vi "_old_Load_SetList_SubVI_v4.1.vi"(0 "Path":path) -> (1 "Procedure Name":string="IBS_PICameraTest_29Sep04", 2 "Paramaters":T1={"Master PB Staging List"=[{"Output Bits"=[], "Delay (s)"="", "String"="", "Halt?"=FALSE}, {"Output Bits"=[], "Delay (s)"="", "String"="", "Halt?"=FALSE}, {"Output Bits"=[], "Delay (s)"="", "String"="", "Halt?"=FALSE}, {"Output Bits"=[], "Delay (s)"="", "String"="", "Halt?"=FALSE}, {"Output Bits"=[], "Delay (s)"="", "String"="", "Halt?"=FALSE}, {"Output Bits"=[], "Delay (s)"="", "String"="", "Halt?"=FALSE}, {"Output Bits"=[], "Delay (s)"="", "String"="", "Halt?"=FALSE}, {"Output Bits"=[], "Delay (s)"="", "String"="", "Halt?"=FALSE}, {"Output Bits"=[], "Delay (s)"="", "String"="", "Halt?"=FALSE}, {"Output Bits"=[], "Delay (s)"="", "String"="", "Halt?"=FALSE}, {"Output Bits"=[], "Delay (s)"="", "String"="", "Halt?"=FALSE}, {"Output Bits"=[], "Delay (s)"="", "String"="", "Halt?"=FALSE}, {"Output Bits"=[], "Delay (s)"="", "String"="", "Halt?"=FALSE}, {"Output Bits"=[], "Delay (s)"="", "String"="", "Halt?"=FALSE}, {"Output Bits"=[], "Delay (s)"="", "String"="", "Halt?"=FALSE}, {"Output Bits"=[], "Delay (s)"="", "String"="", "Halt?"=FALSE}, {"Output Bits"=[], "Delay (s)"="", "String"="", "Halt?"=FALSE}, {"Output Bits"=[], "Delay (s)"="", "String"="", "Halt?"=FALSE}, {"Output Bits"=[], "Delay (s)"="", "String"="", "Halt?"=FALSE}, {"Output Bits"=[], "Delay (s)"="", "String"="", "Halt?"=FALSE}, {"Output Bits"=[], "Delay (s)"="", "String"="", "Halt?"=FALSE}, {"Output Bits"=[], "Delay (s)"="", "String"="", "Halt?"=FALSE}, {"Output Bits"=[], "Delay (s)"="", "String"="", "Halt?"=FALSE}, {"Output Bits"=[], "Delay (s)"="", "String"="", "Halt?"=FALSE}, {"Output Bits"=[], "Delay (s)"="", "String"="", "Halt?"=FALSE}, {"Output Bits"=[], "Delay (s)"="", "String"="", "Halt?"=FALSE}, {"Output Bits"=[], "Delay (s)"="", "String"="", "Halt?"=FALSE}, {"Output Bits"=[], "Delay (s)"="", "String"="", "Halt?"=FALSE}, {"Output Bits"=[], "Delay (s)"="", "String"="", "Halt?"=FALSE}, {"Output Bits"=[], "Delay (s)"="", "String"="", "Halt?"=FALSE}, {"Output Bits"=[], "Delay (s)"="", "String"="", "Halt?"=FALSE}, {"Output Bits"=[], "Delay (s)"="", "String"="", "Halt?"=FALSE}, {"Output Bits"=[], "Delay (s)"="", "String"="", "Halt?"=FALSE}, {"Output Bits"=[], "Delay (s)"="", "String"="", "Halt?"=FALSE}, {"Output Bits"=[], "Delay (s)"="", "String"="", "Halt?"=FALSE}, {"Output Bits"=[], "Delay (s)"="", "String"="", "Halt?"=FALSE}, {"Output Bits"=[], "Delay (s)"="", "String"="", "Halt?"=FALSE}, {"Output Bits"=[], "Delay (s)"="", "String"="", "Halt?"=FALSE}, {"Output Bits"=[], "Delay (s)"="", "String"="", "Halt?"=FALSE}, {"Output Bits"=[], "Delay (s)"="", "String"="", "Halt?"=FALSE}, {"Output Bits"=[], "Delay (s)"="", "String"="", "Halt?"=FALSE}, {"Output Bits"=[], "Delay (s)"="", "String"="", "Halt?"=FALSE}, {"Output Bits"=[], "Delay (s)"="", "String"="", "Halt?"=FALSE}, {"Output Bits"=[], "Delay (s)"="", "String"="", "Halt?"=FALSE}], "Slave PB Staging List"=[{"Output Bits"=[], "Delay (s)"="", "String"="", "Halt?"=FALSE}, {"Output Bits"=[], "Delay (s)"="", "String"="", "Halt?"=FALSE}, {"Output Bits"=[], "Delay (s)"="", "String"="", "Halt?"=FALSE}, {"Output Bits"=[], "Delay (s)"="", "String"="", "Halt?"=FALSE}, {"Output Bits"=[], "Delay (s)"="", "String"="", "Halt?"=FALSE}, {"Output Bits"=[], "Delay (s)"="", "String"="", "Halt?"=FALSE}, {"Output Bits"=[], "Delay (s)"="", "String"="", "Halt?"=FALSE}, {"Output Bits"=[], "Delay (s)"="", "String"="", "Halt?"=FALSE}, {"Output Bits"=[], "Delay (s)"="", "String"="", "Halt?"=FALSE}, {"Output Bits"=[], "Delay (s)"="", "String"="", "Halt?"=FALSE}, {"Output Bits"=[], "Delay (s)"="", "String"="", "Halt?"=FALSE}, {"Output Bits"=[], "Delay (s)"="", "String"="", "Halt?"=FALSE}, {"Output Bits"=[], "Delay (s)"="", "String"="", "Halt?"=FALSE}, {"Output Bits"=[], "Delay (s)"="", "String"="", "Halt?"=FALSE}, {"Output Bits"=[], "Delay (s)"="", "String"="", "Halt?"=FALSE}, {"Output Bits"=[], "Delay (s)"="", "String"="", "Halt?"=FALSE}, {"Output Bits"=[], "Delay (s)"="", "String"="", "Halt?"=FALSE}, {"Output Bits"=[], "Delay (s)"="", "String"="", "Halt?"=FALSE}, {"Output Bits"=[], "Delay (s)"="", "String"="", "Halt?"=FALSE}, {"Output Bits"=[], "Delay (s)"="", "String"="", "Halt?"=FALSE}, {"Output Bits"=[], "Delay (s)"="", "String"="", "Halt?"=FALSE}, {"Output Bits"=[], "Delay (s)"="", "String"="", "Halt?"=FALSE}, {"Output Bits"=[], "Delay (s)"="", "String"="", "Halt?"=FALSE}, {"Output Bits"=[], "Delay (s)"="", "String"="", "Halt?"=FALSE}, {"Output Bits"=[], "Delay (s)"="", "String"="", "Halt?"=FALSE}, {"Output Bits"=[], "Delay (s)"="", "String"="", "Halt?"=FALSE}, {"Output Bits"=[], "Delay (s)"="", "String"="", "Halt?"=FALSE}, {"Output Bits"=[], "Delay (s)"="", "String"="", "Halt?"=FALSE}, {"Output Bits"=[], "Delay (s)"="", "String"="", "Halt?"=FALSE}, {"Output Bits"=[], "Delay (s)"="", "String"="", "Halt?"=FALSE}, {"Output Bits"=[], "Delay (s)"="", "String"="", "Halt?"=FALSE}, {"Output Bits"=[], "Delay (s)"="", "String"="", "Halt?"=FALSE}, {"Output Bits"=[], "Delay (s)"="", "String"="", "Halt?"=FALSE}, {"Output Bits"=[], "Delay (s)"="", "String"="", "Halt?"=FALSE}, {"Output Bits"=[], "Delay (s)"="", "String"="", "Halt?"=FALSE}, {"Output Bits"=[], "Delay (s)"="", "String"="", "Halt?"=FALSE}, {"Output Bits"=[], "Delay (s)"="", "String"="", "Halt?"=FALSE}, {"Output Bits"=[], "Delay (s)"="", "String"="", "Halt?"=FALSE}, {"Output Bits"=[], "Delay (s)"="", "String"="", "Halt?"=FALSE}, {"Output Bits"=[], "Delay (s)"="", "String"="", "Halt?"=FALSE}, {"Output Bits"=[], "Delay (s)"="", "String"="", "Halt?"=FALSE}, {"Output Bits"=[], "Delay (s)"="", "String"="", "Halt?"=FALSE}, {"Output Bits"=[], "Delay (s)"="", "String"="", "Halt?"=FALSE}, {"Output Bits"=[], "Delay (s)"="", "String"="", "Halt?"=FALSE}], "Novatech Ramps"=[{"Ramp Channels"=[], "2 Freq. [MHz]"="", "2 Power [dBm]"="", "3 Freq. [MHz]"="", "3 Power [dBm]"="", "Serial Port"=""}, {"Ramp Channels"=[], "2 Freq. [MHz]"="", "2 Power [dBm]"="", "3 Freq. [MHz]"="", "3 Power [dBm]"="", "Serial Port"=""}, {"Ramp Channels"=[], "2 Freq. [MHz]"="", "2 Power [dBm]"="", "3 Freq. [MHz]"="", "3 Power [dBm]"="", "Serial Port"=""}, {"Ramp Channels"=[], "2 Freq. [MHz]"="", "2 Power [dBm]"="", "3 Freq. [MHz]"="", "3 Power [dBm]"="", "Serial Port"=""}, {"Ramp Channels"=[], "2 Freq. [MHz]"="", "2 Power [dBm]"="", "3 Freq. [MHz]"="", "3 Power [dBm]"="", "Serial Port"=""}, {"Ramp Channels"=[], "2 Freq. [MHz]"="", "2 Power [dBm]"="", "3 Freq. [MHz]"="", "3 Power [dBm]"="", "Serial Port"=""}, {"Ramp Channels"=[], "2 Freq. [MHz]"="", "2 Power [dBm]"="", "3 Freq. [MHz]"="", "3 Power [dBm]"="", "Serial Port"=""}], "Sequencing Info"=[{"Start"=0.0, "End"=2.11, "Sequenced Data"=[], "Inform\nIgor?"=FALSE, "Computed Step Size"=0.0, "Procedure Variable"="", "Default"=2.11, "Steps"=0}], "SRS Ramps"=[{"lattice ramp"=[{"dt"="", "formula"=""}, {"dt"="", "formula"=""}, {"dt"="", "formula"=""}], "Output"=[{"Time Values"=[0.0, 0.002, 0.004, 0.006, 0.008, 0.01, 0.012, 0.014, 0.016, 0.018000000000000002, 0.02, 0.022, 0.024, 0.026000000000000002, 0.028, 0.03, 0.032, 0.034, 0.036000000000000004, 0.038, 0.04, 0.042, 0.044, 0.046, 0.048, 0.05, 0.052000000000000005, 0.054, 0.056, 0.058, 0.06, 0.062, 0.064, 0.066, 0.068, 0.07, 0.07200000000000001, 0.074, 0.076, 0.078, 0.08, 0.082, 0.084, 0.08600000000000001, 0.088, 0.09, 0.092, 0.094, 0.096, 0.098, 0.1, 0.10200000000000001, 0.10400000000000001, 0.106, 0.108, 0.11, 0.112, 0.114, 0.116, 0.11800000000000001, 0.12, 0.122, 0.124, 0.126, 0.128, 0.13, 0.132, 0.134, 0.136, 0.138, 0.14, 0.14200000000000002, 0.14400000000000002, 0.146, 0.148, 0.15, 0.152, 0.154, 0.156, 0.158, 0.16, 0.162, 0.164, 0.166, 0.168, 0.17, 0.17200000000000001, 0.17400000000000002, 0.176, 0.178, 0.18, 0.182, 0.184, 0.186, 0.188, 0.19, 0.192, 0.194, 0.196, 0.198, 0.2, 0.6000000000000001, 0.6000000000000001, 0.6002000000000001, 0.6004, 0.6006000000000001, 0.6008000000000001, 0.6010000000000001, 0.6012000000000001, 0.6014, 0.6016000000000001, 0.6018000000000001, 0.6020000000000001, 0.6022000000000001, 0.6024, 0.6026000000000001, 0.6028000000000001, 0.6030000000000001, 0.6032000000000001, 0.6034, 0.6036000000000001, 0.6038000000000001, 0.6040000000000001, 0.6042000000000001, 0.6044, 0.6046000000000001, 0.6048000000000001, 0.6050000000000001, 0.6052000000000001, 0.6054, 0.6056000000000001, 0.6058000000000001, 0.6060000000000001, 0.6062000000000001, 0.6064, 0.6066000000000001, 0.6068000000000001, 0.6070000000000001, 0.6072000000000001, 0.6074, 0.6076000000000001, 0.6078000000000001, 0.6080000000000001, 0.6082000000000001, 0.6084, 0.6086000000000001, 0.6088000000000001, 0.6090000000000001, 0.6092000000000001, 0.6094, 0.6096000000000001, 0.6098000000000001, 0.6100000000000001, 0.6102000000000001, 0.6104, 0.6106000000000001, 0.6108000000000001, 0.6110000000000001, 0.6112000000000001, 0.6114, 0.6116000000000001, 0.6118000000000001, 0.6120000000000001, 0.6122000000000001, 0.6124, 0.6126, 0.6128000000000001, 0.6130000000000001, 0.6132000000000001, 0.6134000000000001, 0.6136000000000001, 0.6138000000000001, 0.6140000000000001, 0.6142000000000001, 0.6144000000000001, 0.6146, 0.6148000000000001, 0.6150000000000001, 0.6152000000000001, 0.6154000000000001, 0.6156, 0.6158000000000001, 0.6160000000000001, 0.6162000000000001, 0.6164000000000001, 0.6166, 0.6168000000000001, 0.6170000000000001, 0.6172000000000001, 0.6174000000000001, 0.6176, 0.6178000000000001, 0.6180000000000001, 0.6182000000000001, 0.6184000000000001, 0.6186, 0.6188000000000001, 0.6190000000000001, 0.6192000000000001, 0.6194000000000001, 0.6196, 0.6198000000000001, 0.6200000000000001, 0.6202000000000001, 0.6212000000000001], array[205 elements]}, {"Time Values"=[0.0, 0.002, 0.004, 0.006, 0.008, 0.01, 0.012, 0.014, 0.016, 0.018000000000000002, 0.02, 0.022, 0.024, 0.026000000000000002, 0.028, 0.03, 0.032, 0.034, 0.036000000000000004, 0.038, 0.04, 0.042, 0.044, 0.046, 0.048, 0.05, 0.052000000000000005, 0.054, 0.056, 0.058, 0.06, 0.062, 0.064, 0.066, 0.068, 0.07, 0.07200000000000001, 0.074, 0.076, 0.078, 0.08, 0.082, 0.084, 0.08600000000000001, 0.088, 0.09, 0.092, 0.094, 0.096, 0.098, 0.1, 0.10200000000000001, 0.10400000000000001, 0.106, 0.108, 0.11, 0.112, 0.114, 0.116, 0.11800000000000001, 0.12, 0.122, 0.124, 0.126, 0.128, 0.13, 0.132, 0.134, 0.136, 0.138, 0.14, 0.14200000000000002, 0.14400000000000002, 0.146, 0.148, 0.15, 0.152, 0.154, 0.156, 0.158, 0.16, 0.162, 0.164, 0.166, 0.168, 0.17, 0.17200000000000001, 0.17400000000000002, 0.176, 0.178, 0.18, 0.182, 0.184, 0.186, 0.188, 0.19, 0.192, 0.194, 0.196, 0.198, 0.2, 0.6000000000000001, 0.6000000000000001, 0.6002000000000001, 0.6004, 0.6006000000000001, 0.6008000000000001, 0.6010000000000001, 0.6012000000000001, 0.6014, 0.6016000000000001, 0.6018000000000001, 0.6020000000000001, 0.6022000000000001, 0.6024, 0.6026000000000001, 0.6028000000000001, 0.6030000000000001, 0.6032000000000001, 0.6034, 0.6036000000000001, 0.6038000000000001, 0.6040000000000001, 0.6042000000000001, 0.6044, 0.6046000000000001, 0.6048000000000001, 0.6050000000000001, 0.6052000000000001, 0.6054, 0.6056000000000001, 0.6058000000000001, 0.6060000000000001, 0.6062000000000001, 0.6064, 0.6066000000000001, 0.6068000000000001, 0.6070000000000001, 0.6072000000000001, 0.6074, 0.6076000000000001, 0.6078000000000001, 0.6080000000000001, 0.6082000000000001, 0.6084, 0.6086000000000001, 0.6088000000000001, 0.6090000000000001, 0.6092000000000001, 0.6094, 0.6096000000000001, 0.6098000000000001, 0.6100000000000001, 0.6102000000000001, 0.6104, 0.6106000000000001, 0.6108000000000001, 0.6110000000000001, 0.6112000000000001, 0.6114, 0.6116000000000001, 0.6118000000000001, 0.6120000000000001, 0.6122000000000001, 0.6124, 0.6126, 0.6128000000000001, 0.6130000000000001, 0.6132000000000001, 0.6134000000000001, 0.6136000000000001, 0.6138000000000001, 0.6140000000000001, 0.6142000000000001, 0.6144000000000001, 0.6146, 0.6148000000000001, 0.6150000000000001, 0.6152000000000001, 0.6154000000000001, 0.6156, 0.6158000000000001, 0.6160000000000001, 0.6162000000000001, 0.6164000000000001, 0.6166, 0.6168000000000001, 0.6170000000000001, 0.6172000000000001, 0.6174000000000001, 0.6176, 0.6178000000000001, 0.6180000000000001, 0.6182000000000001, 0.6184000000000001, 0.6186, 0.6188000000000001, 0.6190000000000001, 0.6192000000000001, 0.6194000000000001, 0.6196, 0.6198000000000001, 0.6200000000000001, 0.6202000000000001, 0.6212000000000001], array[205 elements]}], "SRS Selection"=enum."1550 Vertical"}, {"lattice ramp"=[{"dt"="", "formula"=""}], "Output"=[{"Time Values"=[0.0, 0.002, 0.004, 0.006, 0.008, 0.01, 0.012, 0.014, 0.016, 0.018000000000000002, 0.02, 0.022, 0.024, 0.026000000000000002, 0.028, 0.03, 0.032, 0.034, 0.036000000000000004, 0.038, 0.04, 0.042, 0.044, 0.046, 0.048, 0.05, 0.052000000000000005, 0.054, 0.056, 0.058, 0.06, 0.062, 0.064, 0.066, 0.068, 0.07, 0.07200000000000001, 0.074, 0.076, 0.078, 0.08, 0.082, 0.084, 0.08600000000000001, 0.088, 0.09, 0.092, 0.094, 0.096, 0.098, 0.1, 0.10200000000000001, 0.10400000000000001, 0.106, 0.108, 0.11, 0.112, 0.114, 0.116, 0.11800000000000001, 0.12, 0.122, 0.124, 0.126, 0.128, 0.13, 0.132, 0.134, 0.136, 0.138, 0.14, 0.14200000000000002, 0.14400000000000002, 0.146, 0.148, 0.15, 0.152, 0.154, 0.156, 0.158, 0.16, 0.162, 0.164, 0.166, 0.168, 0.17, 0.17200000000000001, 0.17400000000000002, 0.176, 0.178, 0.18, 0.182, 0.184, 0.186, 0.188, 0.19, 0.192, 0.194, 0.196, 0.198, 0.2, 0.6000000000000001, 0.6000000000000001, 0.6002000000000001, 0.6004, 0.6006000000000001, 0.6008000000000001, 0.6010000000000001, 0.6012000000000001, 0.6014, 0.6016000000000001, 0.6018000000000001, 0.6020000000000001, 0.6022000000000001, 0.6024, 0.6026000000000001, 0.6028000000000001, 0.6030000000000001, 0.6032000000000001, 0.6034, 0.6036000000000001, 0.6038000000000001, 0.6040000000000001, 0.6042000000000001, 0.6044, 0.6046000000000001, 0.6048000000000001, 0.6050000000000001, 0.6052000000000001, 0.6054, 0.6056000000000001, 0.6058000000000001, 0.6060000000000001, 0.6062000000000001, 0.6064, 0.6066000000000001, 0.6068000000000001, 0.6070000000000001, 0.6072000000000001, 0.6074, 0.6076000000000001, 0.6078000000000001, 0.6080000000000001, 0.6082000000000001, 0.6084, 0.6086000000000001, 0.6088000000000001, 0.6090000000000001, 0.6092000000000001, 0.6094, 0.6096000000000001, 0.6098000000000001, 0.6100000000000001, 0.6102000000000001, 0.6104, 0.6106000000000001, 0.6108000000000001, 0.6110000000000001, 0.6112000000000001, 0.6114, 0.6116000000000001, 0.6118000000000001, 0.6120000000000001, 0.6122000000000001, 0.6124, 0.6126, 0.6128000000000001, 0.6130000000000001, 0.6132000000000001, 0.6134000000000001, 0.6136000000000001, 0.6138000000000001, 0.6140000000000001, 0.6142000000000001, 0.6144000000000001, 0.6146, 0.6148000000000001, 0.6150000000000001, 0.6152000000000001, 0.6154000000000001, 0.6156, 0.6158000000000001, 0.6160000000000001, 0.6162000000000001, 0.6164000000000001, 0.6166, 0.6168000000000001, 0.6170000000000001, 0.6172000000000001, 0.6174000000000001, 0.6176, 0.6178000000000001, 0.6180000000000001, 0.6182000000000001, 0.6184000000000001, 0.6186, 0.6188000000000001, 0.6190000000000001, 0.6192000000000001, 0.6194000000000001, 0.6196, 0.6198000000000001, 0.6200000000000001, 0.6202000000000001, 0.6212000000000001], array[205 elements]}, {"Time Values"=[0.0, 0.002, 0.004, 0.006, 0.008, 0.01, 0.012, 0.014, 0.016, 0.018000000000000002, 0.02, 0.022, 0.024, 0.026000000000000002, 0.028, 0.03, 0.032, 0.034, 0.036000000000000004, 0.038, 0.04, 0.042, 0.044, 0.046, 0.048, 0.05, 0.052000000000000005, 0.054, 0.056, 0.058, 0.06, 0.062, 0.064, 0.066, 0.068, 0.07, 0.07200000000000001, 0.074, 0.076, 0.078, 0.08, 0.082, 0.084, 0.08600000000000001, 0.088, 0.09, 0.092, 0.094, 0.096, 0.098, 0.1, 0.10200000000000001, 0.10400000000000001, 0.106, 0.108, 0.11, 0.112, 0.114, 0.116, 0.11800000000000001, 0.12, 0.122, 0.124, 0.126, 0.128, 0.13, 0.132, 0.134, 0.136, 0.138, 0.14, 0.14200000000000002, 0.14400000000000002, 0.146, 0.148, 0.15, 0.152, 0.154, 0.156, 0.158, 0.16, 0.162, 0.164, 0.166, 0.168, 0.17, 0.17200000000000001, 0.17400000000000002, 0.176, 0.178, 0.18, 0.182, 0.184, 0.186, 0.188, 0.19, 0.192, 0.194, 0.196, 0.198, 0.2, 0.6000000000000001, 0.6000000000000001, 0.6002000000000001, 0.6004, 0.6006000000000001, 0.6008000000000001, 0.6010000000000001, 0.6012000000000001, 0.6014, 0.6016000000000001, 0.6018000000000001, 0.6020000000000001, 0.6022000000000001, 0.6024, 0.6026000000000001, 0.6028000000000001, 0.6030000000000001, 0.6032000000000001, 0.6034, 0.6036000000000001, 0.6038000000000001, 0.6040000000000001, 0.6042000000000001, 0.6044, 0.6046000000000001, 0.6048000000000001, 0.6050000000000001, 0.6052000000000001, 0.6054, 0.6056000000000001, 0.6058000000000001, 0.6060000000000001, 0.6062000000000001, 0.6064, 0.6066000000000001, 0.6068000000000001, 0.6070000000000001, 0.6072000000000001, 0.6074, 0.6076000000000001, 0.6078000000000001, 0.6080000000000001, 0.6082000000000001, 0.6084, 0.6086000000000001, 0.6088000000000001, 0.6090000000000001, 0.6092000000000001, 0.6094, 0.6096000000000001, 0.6098000000000001, 0.6100000000000001, 0.6102000000000001, 0.6104, 0.6106000000000001, 0.6108000000000001, 0.6110000000000001, 0.6112000000000001, 0.6114, 0.6116000000000001, 0.6118000000000001, 0.6120000000000001, 0.6122000000000001, 0.6124, 0.6126, 0.6128000000000001, 0.6130000000000001, 0.6132000000000001, 0.6134000000000001, 0.6136000000000001, 0.6138000000000001, 0.6140000000000001, 0.6142000000000001, 0.6144000000000001, 0.6146, 0.6148000000000001, 0.6150000000000001, 0.6152000000000001, 0.6154000000000001, 0.6156, 0.6158000000000001, 0.6160000000000001, 0.6162000000000001, 0.6164000000000001, 0.6166, 0.6168000000000001, 0.6170000000000001, 0.6172000000000001, 0.6174000000000001, 0.6176, 0.6178000000000001, 0.6180000000000001, 0.6182000000000001, 0.6184000000000001, 0.6186, 0.6188000000000001, 0.6190000000000001, 0.6192000000000001, 0.6194000000000001, 0.6196, 0.6198000000000001, 0.6200000000000001, 0.6202000000000001, 0.6212000000000001], array[205 elements]}], "SRS Selection"=enum."1550 Vertical"}], "Master AO Ramp List"=[{"Ramp index"=10, "Ramp time [s]"="", "Step size [s]"=1000.0, "Ramp Array"=[], "Output Bits"=[]}, {"Ramp index"=10, "Ramp time [s]"="", "Step size [s]"=1000.0, "Ramp Array"=[], "Output Bits"=[]}], "Slave AO Ramp List"=[{"Ramp index"=10, "Ramp time [s]"="", "Step size [s]"=1000.0, "Ramp Array"=[], "Output Bits"=[]}, {"Ramp index"=10, "Ramp time [s]"="", "Step size [s]"=1000.0, "Ramp Array"=[], "Output Bits"=[]}], "Master Novatech Ramp List"=[], "Static Variables"=[], "DDS Ramp List"=[]} {"Sequencing Info"."Steps" min=2; "Sequencing Info"."Default" format="%#.7p"; "Sequencing Info"."Computed Step Size" format="%#.7p"; "Sequencing Info"."Sequenced Data" format="%.2e"; "Sequencing Info"."End" format="%#.7p"; "Sequencing Info"."Start" format="%#.7p"})   [LabVIEW 2013]
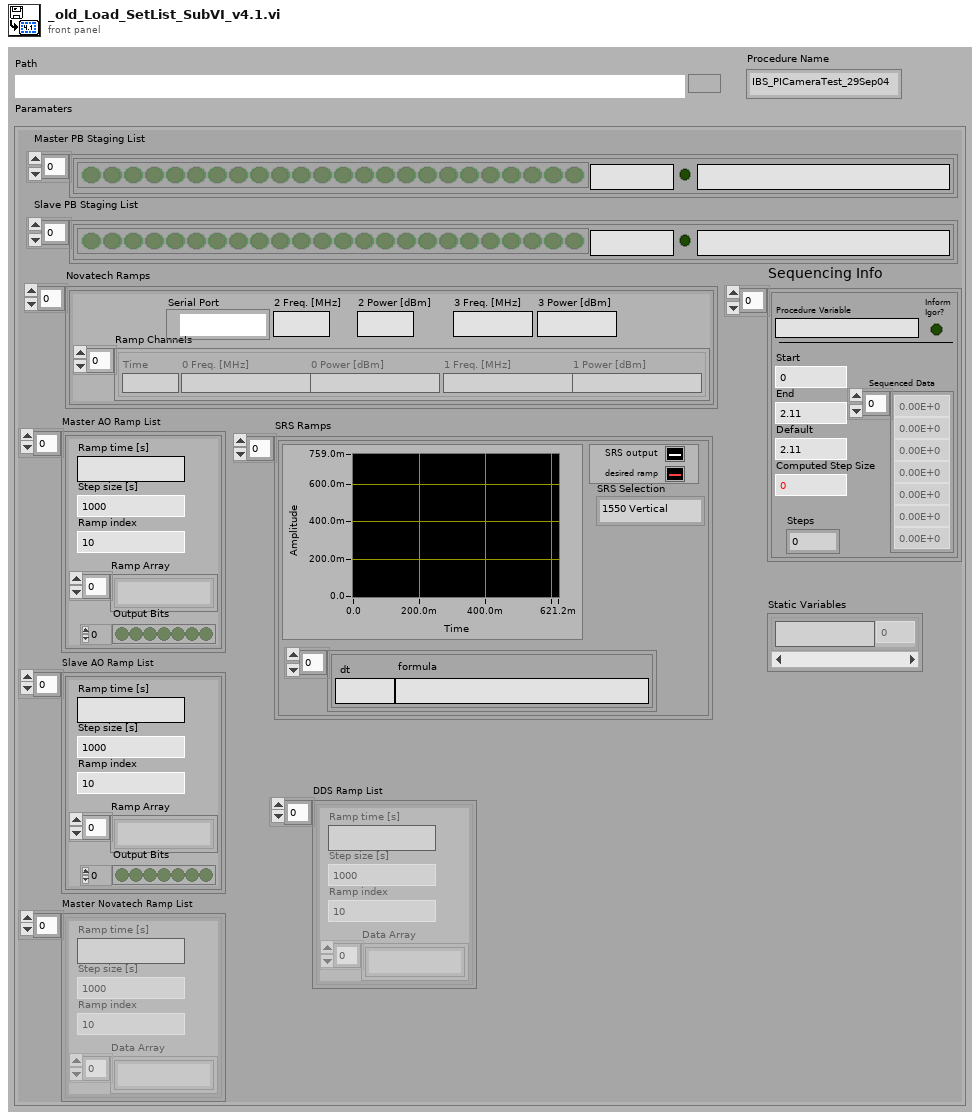
[diagram p1: front panel]
types:
  T1 = cluster{"Master PB Staging List":cluster{"Output Bits":bool[], "Delay (s)":string, "String":string, "Halt?":bool}[], "Slave PB Staging List":cluster{"Output Bits":bool[], "Delay (s)":string, "String":string, "Halt?":bool}[], "Novatech Ramps":cluster{"Ramp Channels":cluster{"Time":string, "0 Freq. [MHz]":string, "0 Power [dBm]":string, "1 Freq. [MHz]":string, "1 Power [dBm]":string}[], "2 Freq. [MHz]":string, "2 Power [dBm]":string, "3 Freq. [MHz]":string, "3 Power [dBm]":string, "Serial Port":refnum<visa-resource-name>}[], "Sequencing Info":cluster{"Start":dbl, "End":dbl, "Sequenced Data":dbl[], "Inform\nIgor?":bool, "Computed Step Size":dbl, "Procedure Variable":string, "Default":dbl, "Steps":i32}[], "SRS Ramps":cluster{"lattice ramp":cluster{"dt":string, "formula":string}[], "Output":cluster{"Time Values":dbl[], dbl[]}[], "SRS Selection":enum16{"1550 Vertical", "Bragg Agilent", "Bragg PTS", "Acc. Intensity"}}[], "Master AO Ramp List":cluster{"Ramp index":u32, "Ramp time [s]":string, "Step size [s]":dbl, "Ramp Array":string[], "Output Bits":bool[]}[], "Slave AO Ramp List":cluster{"Ramp index":u32, "Ramp time [s]":string, "Step size [s]":dbl, "Ramp Array":string[], "Output Bits":bool[]}[], "Master Novatech Ramp List":cluster{"Ramp index":u32, "Ramp time [s]":string, "Step size [s]":dbl, "Data Array":string[]}[], "Static Variables":cluster{"Procedure variable":string, "Value":dbl}[], "DDS Ramp List":cluster{"Ramp index":u32, "Ramp time [s]":string, "Step size [s]":dbl, "Data Array":string[]}[]}
  T2 = cluster{"Output Bits":bool[], "Delay (s)":string, "String":string, "Halt?":bool}[]
  T3 = cluster{"Ramp index":u32, "Ramp time [s]":string, "Step size [s]":dbl, "Ramp Array":string[], "Output Bits":bool[]}[]
  T4 = cluster{"Ramp index":u32, "Ramp time [s]":string, "Step size [s]":dbl, "Data Array":string[]}[]
  T5 = cluster{"Ramp Channels":cluster{"Time":string, "0 Freq. [MHz]":string, "0 Power [dBm]":string, "1 Freq. [MHz]":string, "1 Power [dBm]":string}[], "2 Freq. [MHz]":string, "2 Power [dBm]":string, "3 Freq. [MHz]":string, "3 Power [dBm]":string, "Serial Port":refnum<visa-resource-name>}[]
  T6 = cluster{"Start":dbl, "End":dbl, "Sequenced Data":dbl[], "Inform\nIgor?":bool, "Computed Step Size":dbl, "Procedure Variable":string, "Default":dbl, "Steps":i32}[]
  T7 = cluster{"lattice ramp":cluster{"dt":string, "formula":string}[], "Output":cluster{"Time Values":dbl[], dbl[]}[], "SRS Selection":enum16{"1550 Vertical", "Bragg Agilent", "Bragg PTS", "Acc. Intensity"}}[]
  T8 = cluster{"Procedure variable":string, "Value":dbl}[]
  T9 = cluster{"Ramp index":u32, "Ramp time [s]":string, "Step size [s]":dbl, "Ramp Array":string[], "Output Bits":bool[]}
  T10 = cluster{"Ramp index":u32, "Ramp time [s]":string, "Step size [s]":dbl, "Data Array":string[]}
  T11 = cluster{"Output Bits":bool[], "Delay (s)":string, "String":string, "Halt?":bool}
  T12 = cluster{"Ramp Channels":cluster{"Time":string, "0 Freq. [MHz]":string, "0 Power [dBm]":string, "1 Freq. [MHz]":string, "1 Power [dBm]":string}[], "2 Freq. [MHz]":string, "2 Power [dBm]":string, "3 Freq. [MHz]":string, "3 Power [dBm]":string, "Serial Port":refnum<visa-resource-name>}
  T13 = cluster{"Start":dbl, "End":dbl, "Sequenced Data":dbl[], "Inform\nIgor?":bool, "Computed Step Size":dbl, "Procedure Variable":string, "Default":dbl, "Steps":i32}
  T14 = cluster{"Procedure variable":string, "Value":dbl}
  T15 = cluster{"lattice ramp":cluster{"dt":string, "formula":string}[], "Output":cluster{"Time Values":dbl[], dbl[]}[], "SRS Selection":enum16{"1550 Vertical", "Bragg Agilent", "Bragg PTS", "Acc. Intensity"}}
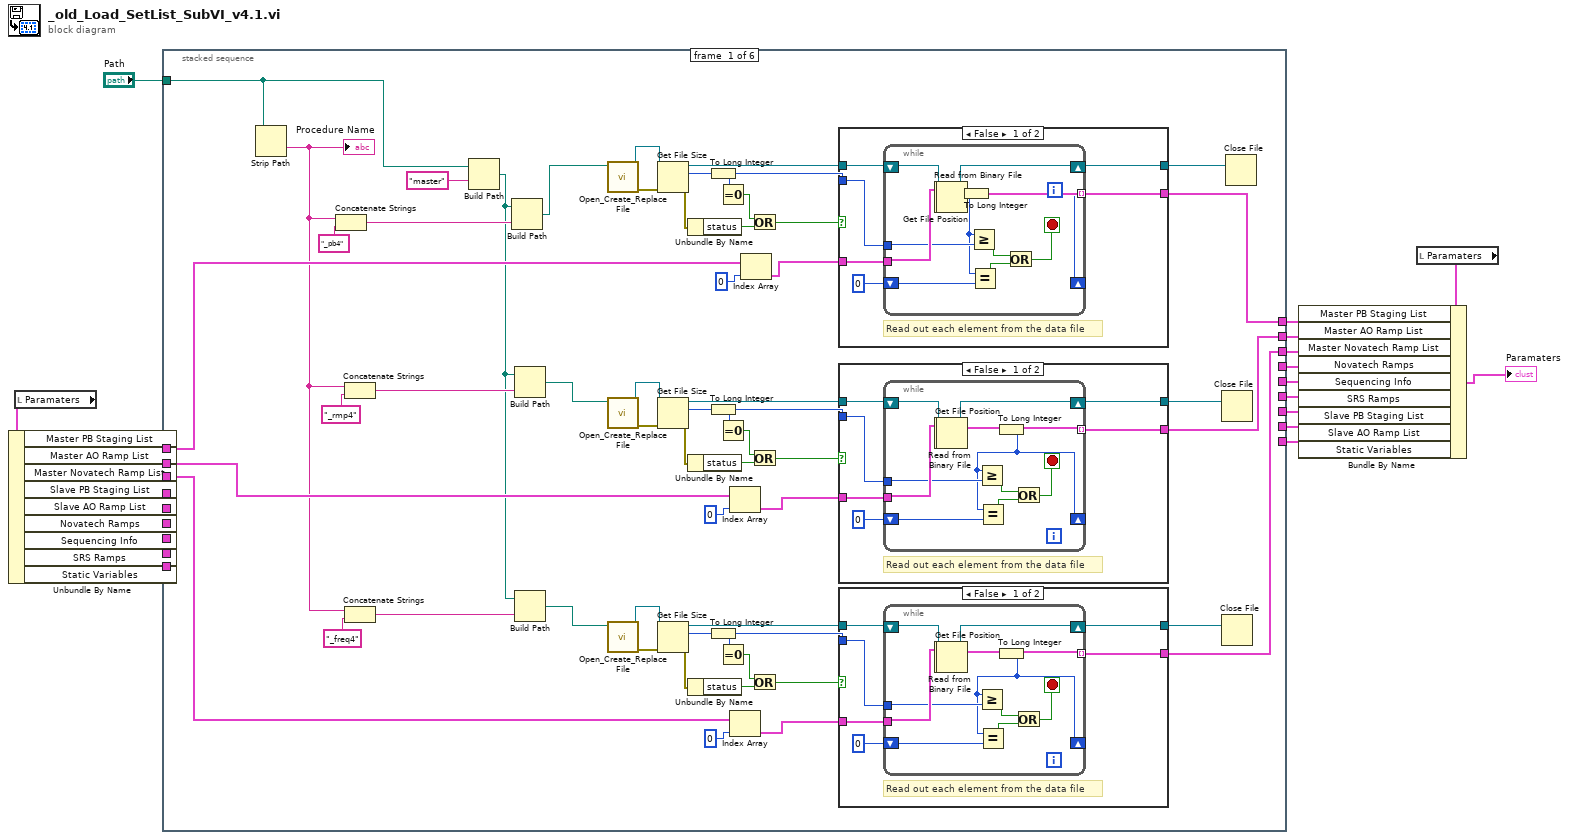
[diagram p0: block diagram]
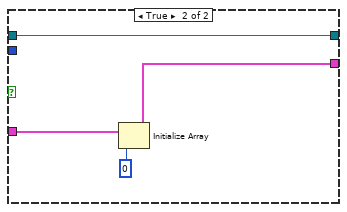
[diagram p2: hidden frame]
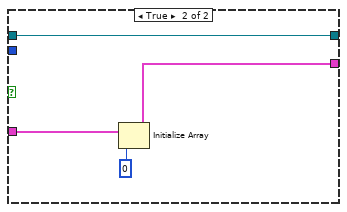
[diagram p3: hidden frame]
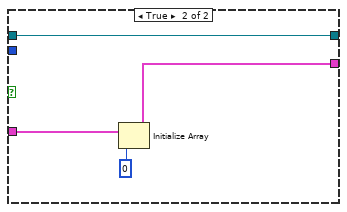
[diagram p4: hidden frame]
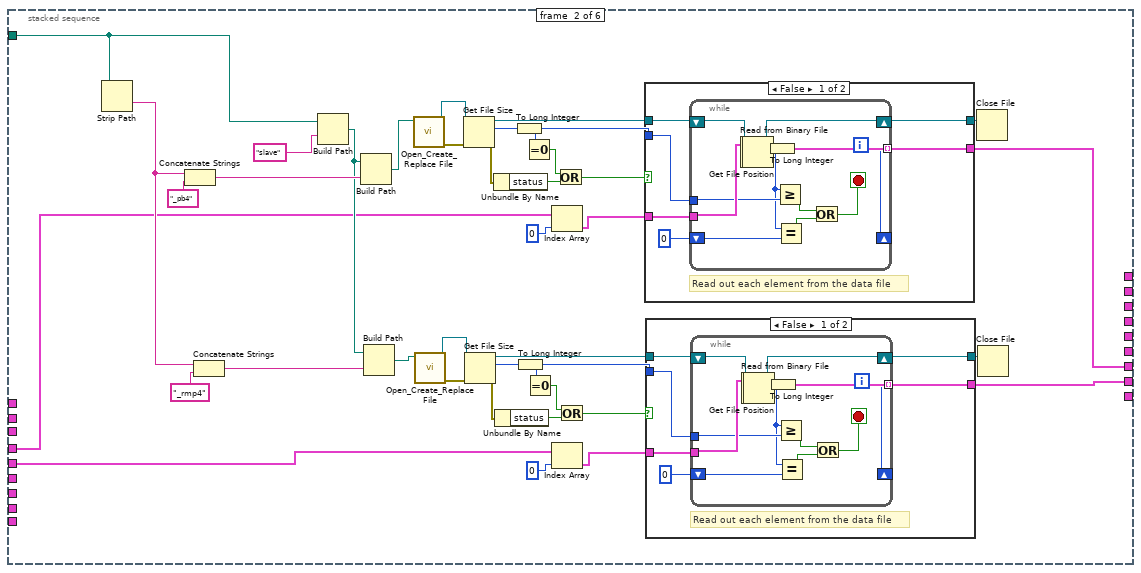
[diagram p5: hidden frame]
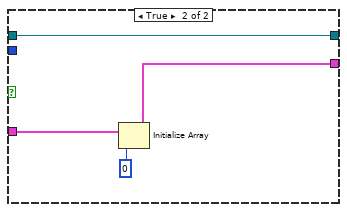
[diagram p6: hidden frame]
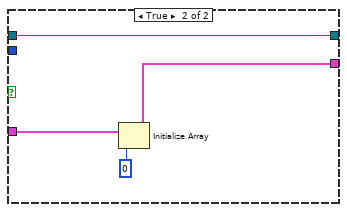
[diagram p7: hidden frame]
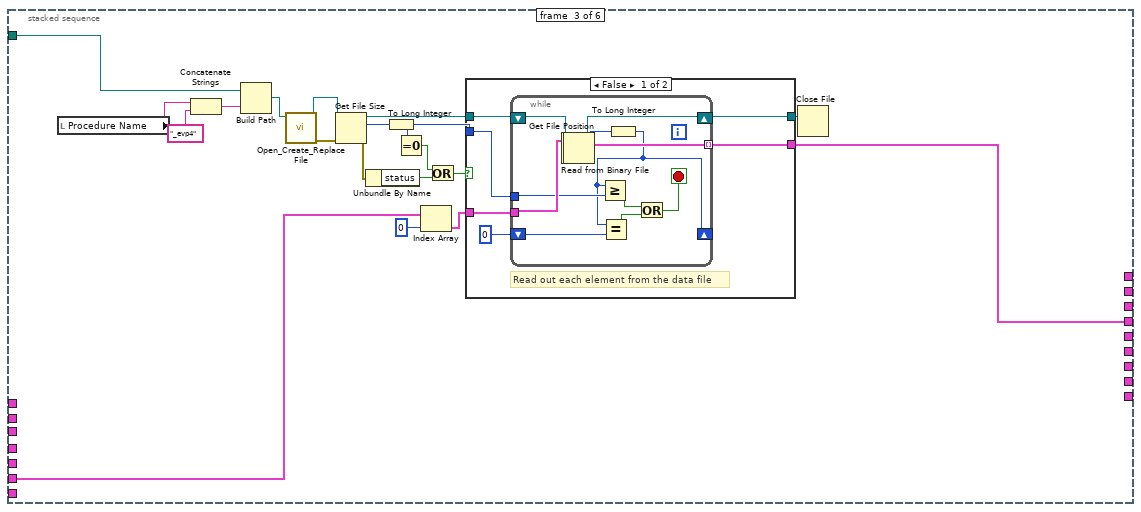
[diagram p8: hidden frame]
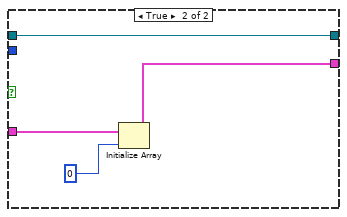
[diagram p9: hidden frame]
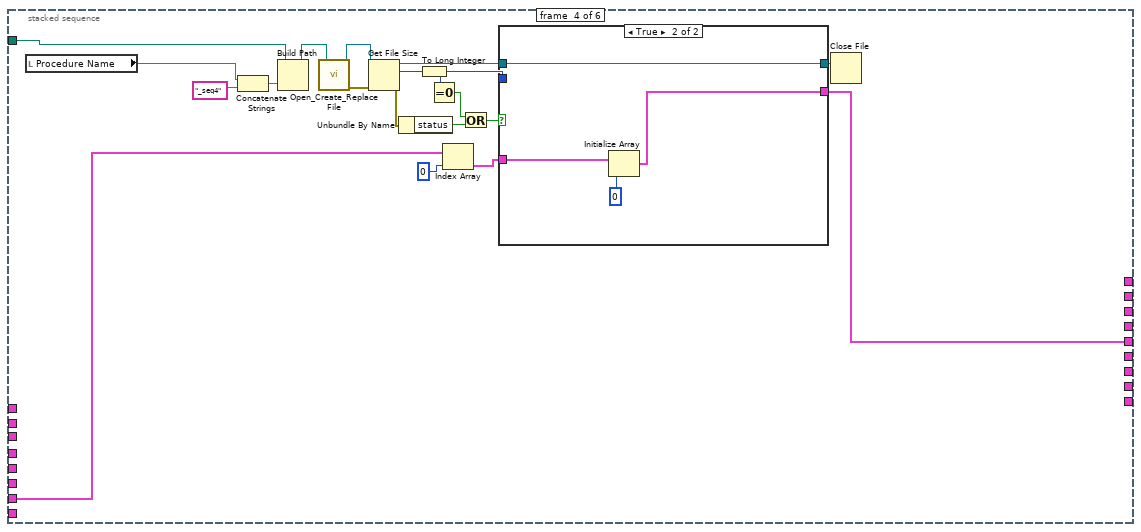
[diagram p10: hidden frame]
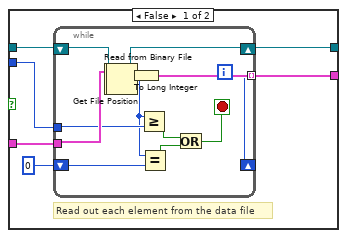
[diagram p11: hidden frame]
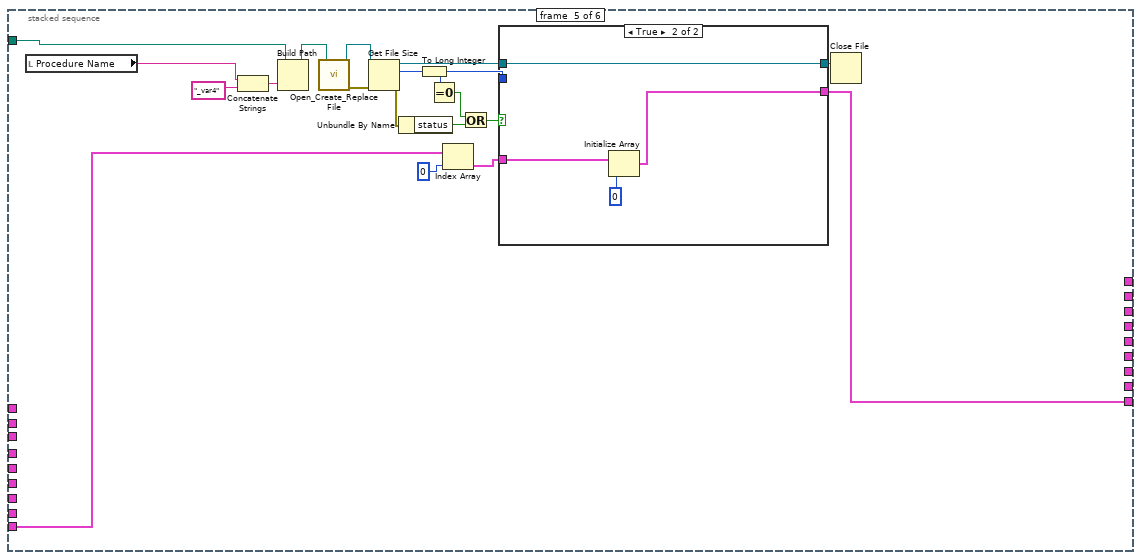
[diagram p12: hidden frame]
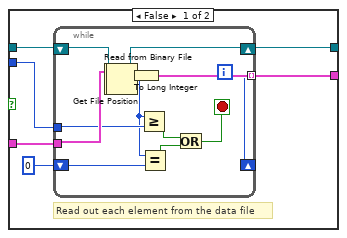
[diagram p13: hidden frame]
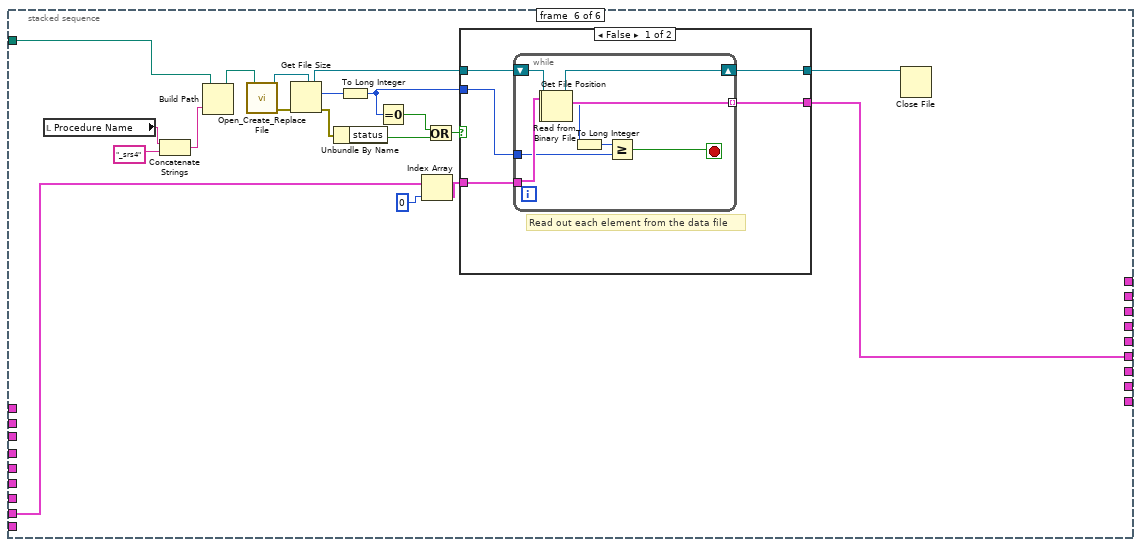
[diagram p14: hidden frame]
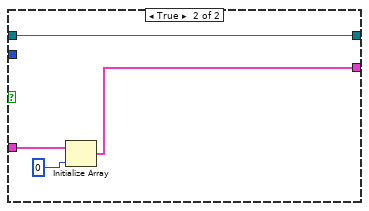
[diagram p15: hidden frame]
diagram:
  n1 = local read "Paramaters"() -> (w20:T1)
  n2 = Unbundle By Name(w20) -> ("Master PB Staging List"=w19:T2, "Master AO Ramp List"=w18:T3, "Master Novatech Ramp List"=w3:T4, "Slave PB Staging List"=w17:T2, "Slave AO Ramp List"=w16:T3, "Novatech Ramps"=w15:T5, "Sequencing Info"=w14:T6, "SRS Ramps"=w13:T7, "Static Variables"=w2:T8)
  n3 = stacked-sequence {
    tunnel: [_ _ _ _ _ w369] -> w5
    tunnel: [_ _ _ w284 _ _] -> w6
    tunnel: w19 -> [w46 _ _ _ _ _]
    tunnel: w18 -> [w42 _ _ _ _ _]
    tunnel: w17 -> [_ w150 _ _ _ _]
    tunnel: w16 -> [_ w147 _ _ _ _]
    tunnel: w15 -> [_ _ w236 _ _ _]
    tunnel: w14 -> [_ _ _ w273 _ _]
    tunnel: w13 -> [_ _ _ _ _ w357]
    tunnel: [w62 _ _ _ _ _] -> w12
    tunnel: "Path" -> [w51 w167 w234 w276 w319 w360]
    tunnel: [w50 _ _ _ _ _] -> w10
    tunnel: [_ _ w231 _ _ _] -> w7
    tunnel: [_ w166 _ _ _ _] -> w9
    tunnel: [_ w155 _ _ _ _] -> w8
    tunnel: [w23 _ _ _ _ _] -> w4
    tunnel: w3 -> [w24 _ _ _ _ _]
    tunnel: w2 -> [_ _ _ _ w316 _]
    tunnel: [_ _ _ _ w315 _] -> w1
    frame #0 {
      n4 = Strip Path(path=w51) -> (name=w26:string)  [unwired: 1 out]
      "Procedure Name" <- w26
      n5 = Concatenate Strings(w26, "_pb4") -> (w75:string)
      n6 = Concatenate Strings(w26, "_rmp4") -> (w73:string)
      n7 = Concatenate Strings(w26, "_freq4") -> (w40:string)
      n8 = Build Path(base path=w51, name or relative path="master") -> (appended path=w25:path)
      n9 = Build Path(base path=w25, name or relative path=w75) -> (appended path=w49:path)
      n10 = Build Path(base path=w25, name or relative path=w73) -> (appended path=w48:path)
      n11 = Build Path(base path=w25, name or relative path=w40) -> (appended path=w29:path)
      n12 = call <vilib>:"Open_Create_Replace File.vi"("file path"=w49) -> ("error out"=w64:errorcluster, "refnum"=w71:refnum<file>)  [unwired: 5 in, 4 out]
      n13 = call <vilib>:"Open_Create_Replace File.vi"("file path"=w48) -> ("error out"=w53:errorcluster, "refnum"=w60:refnum<file>)  [unwired: 5 in, 4 out]
      n14 = call <vilib>:"Open_Create_Replace File.vi"("file path"=w29) -> ("error out"=w31:errorcluster, "refnum"=w38:refnum<file>)  [unwired: 5 in, 4 out]
      n15 = Get File Size(file=w71, error in=w64) -> (refnum out=w70:refnum<file>, size (in bytes)=w68:i64, 0:w63:errorcluster)
      n16 = Get File Size(file=w60, error in=w53) -> (refnum out=w59:refnum<file>, size (in bytes)=w57:i64, 0:w52:errorcluster)
      n17 = Get File Size(file=w38, error in=w31) -> (refnum out=w37:refnum<file>, size (in bytes)=w35:i64, 0:w30:errorcluster)
      n18 = Unbundle By Name(w63) -> ("status"=w65:bool)
      n19 = Unbundle By Name(w52) -> ("status"=w54:bool)
      n20 = Unbundle By Name(w30) -> ("status"=w32:bool)
      n21 = To Long Integer(number=w68) -> (32bit integer=w69:i32)
      n22 = To Long Integer(number=w57) -> (32bit integer=w58:i32)
      n23 = To Long Integer(number=w35) -> (32bit integer=w36:i32)
      n24 = Equal To 0?(x=w69) -> (x = 0?=w66:bool)
      n25 = Equal To 0?(x=w58) -> (x = 0?=w55:bool)
      n26 = Equal To 0?(x=w36) -> (x = 0?=w33:bool)
      n27 = Index Array(array=w42, index=0) -> (element=w43:T9)
      n28 = Index Array(array=w24, index=0) -> (element=w27:T10)
      n29 = Index Array(array=w46, index=0) -> (element=w45:T11)
      n30 = Or(x=w66, y=w65) -> (x .or. y?=w67:bool)
      n31 = Or(x=w55, y=w54) -> (x .or. y?=w56:bool)
      n32 = Or(x=w33, y=w32) -> (x .or. y?=w34:bool)
      n33 = case shown="False" w67 {
        tunnel: [w129 w146] -> w72
        tunnel: w45 -> [w128 w144]
        tunnel: w70 -> [w127 w146]
        tunnel: [w126 w145] -> w62
        tunnel: w69 -> [w125 _]
        frame False {
          # "Read out each element from the data file"
          n34 = while {
            tunnel: [w140] -> w126 mode=indexing
            tunnel: w128 -> [w139]
            shift-right: [w141] -> w129
            shift-left: w127 -> [w142]
            tunnel: w125 -> [w138]
            shift-right: [w137] -> _
            shift-left: 0 -> [w136]
            stop <- w133 stop-if-true
            n35 = Read from Binary File(5:w139, 11:w142) -> (0:w131:errorcluster, 2:w140:T11, 3:w132:refnum<file>)  [unwired: 1 in, 4 out]
            n36 = Get File Position(4:w131, 7:w132) -> (2:w130:i64, 3:w141:refnum<file>)  [unwired: 1 out]
            n37 = To Long Integer(number=w130) -> (32bit integer=w137:i32)
            n38 = Greater Or Equal?(x=w137, y=w138) -> (x >= y?=w134:bool)
            n39 = Equal?(x=w137, y=w136) -> (x = y?=w135:bool)
            n40 = Or(x=w134, y=w135) -> (x .or. y?=w133:bool)
          }
        }
        frame True {
          n41 = Initialize Array(w144, 0) -> (w145:T2)
        }
      }
      n42 = case shown="False" w56 {
        tunnel: [w106 w123] -> w61
        tunnel: w43 -> [w105 w121]
        tunnel: w59 -> [w104 w123]
        tunnel: [w103 w122] -> w50
        tunnel: w58 -> [w102 _]
        frame False {
          # "Read out each element from the data file"
          n43 = while {
            tunnel: [w117] -> w103 mode=indexing
            tunnel: w105 -> [w116]
            shift-right: [w118] -> w106
            shift-left: w104 -> [w119]
            tunnel: w102 -> [w115]
            shift-right: [w114] -> _
            shift-left: 0 -> [w113]
            stop <- w110 stop-if-true
            n44 = Read from Binary File(5:w116, 11:w119) -> (0:w108:errorcluster, 2:w117:T9, 3:w109:refnum<file>)  [unwired: 1 in, 4 out]
            n45 = Get File Position(4:w108, 7:w109) -> (2:w107:i64, 3:w118:refnum<file>)  [unwired: 1 out]
            n46 = To Long Integer(number=w107) -> (32bit integer=w114:i32)
            n47 = Greater Or Equal?(x=w114, y=w115) -> (x >= y?=w111:bool)
            n48 = Equal?(x=w114, y=w113) -> (x = y?=w112:bool)
            n49 = Or(x=w111, y=w112) -> (x .or. y?=w110:bool)
          }
        }
        frame True {
          n50 = Initialize Array(w121, 0) -> (w122:T3)
        }
      }
      n51 = case shown="False" w34 {
        tunnel: [w83 w100] -> w39
        tunnel: w27 -> [w82 w98]
        tunnel: w37 -> [w81 w100]
        tunnel: [w80 w99] -> w23
        tunnel: w36 -> [w79 _]
        frame False {
          # "Read out each element from the data file"
          n52 = while {
            tunnel: [w94] -> w80 mode=indexing
            tunnel: w82 -> [w93]
            shift-right: [w95] -> w83
            shift-left: w81 -> [w96]
            tunnel: w79 -> [w92]
            shift-right: [w91] -> _
            shift-left: 0 -> [w90]
            stop <- w87 stop-if-true
            n53 = Read from Binary File(5:w93, 11:w96) -> (0:w85:errorcluster, 2:w94:T10, 3:w86:refnum<file>)  [unwired: 1 in, 4 out]
            n54 = Get File Position(4:w85, 7:w86) -> (2:w84:i64, 3:w95:refnum<file>)  [unwired: 1 out]
            n55 = To Long Integer(number=w84) -> (32bit integer=w91:i32)
            n56 = Greater Or Equal?(x=w91, y=w92) -> (x >= y?=w88:bool)
            n57 = Equal?(x=w91, y=w90) -> (x = y?=w89:bool)
            n58 = Or(x=w88, y=w89) -> (x .or. y?=w87:bool)
          }
        }
        frame True {
          n59 = Initialize Array(w98, 0) -> (w99:T4)
        }
      }
      n60 = Close File(refnum=w61) -> ()  [unwired: 1 in, 2 out]
      n61 = Close File(refnum=w39) -> ()  [unwired: 1 in, 2 out]
      n62 = Close File(refnum=w72) -> ()  [unwired: 1 in, 2 out]
    }
    frame #1 {
      n63 = Strip Path(path=w167) -> (name=w178:string)  [unwired: 1 out]
      n64 = Concatenate Strings(w178, "_pb4") -> (w182:string)
      n65 = Concatenate Strings(w178, "_rmp4") -> (w180:string)
      n66 = Build Path(base path=w167, name or relative path="slave") -> (appended path=w179:path)
      n67 = Build Path(base path=w179, name or relative path=w182) -> (appended path=w154:path)
      n68 = Build Path(base path=w179, name or relative path=w180) -> (appended path=w153:path)
      n69 = call <vilib>:"Open_Create_Replace File.vi"("file path"=w154) -> ("error out"=w169:errorcluster, "refnum"=w176:refnum<file>)  [unwired: 5 in, 4 out]
      n70 = call <vilib>:"Open_Create_Replace File.vi"("file path"=w153) -> ("error out"=w157:errorcluster, "refnum"=w164:refnum<file>)  [unwired: 5 in, 4 out]
      n71 = Get File Size(file=w176, error in=w169) -> (refnum out=w175:refnum<file>, size (in bytes)=w173:i64, 0:w168:errorcluster)
      n72 = Get File Size(file=w164, error in=w157) -> (refnum out=w163:refnum<file>, size (in bytes)=w161:i64, 0:w156:errorcluster)
      n73 = Unbundle By Name(w168) -> ("status"=w170:bool)
      n74 = Unbundle By Name(w156) -> ("status"=w158:bool)
      n75 = To Long Integer(number=w173) -> (32bit integer=w174:i32)
      n76 = To Long Integer(number=w161) -> (32bit integer=w162:i32)
      n77 = Equal To 0?(x=w174) -> (x = 0?=w171:bool)
      n78 = Equal To 0?(x=w162) -> (x = 0?=w159:bool)
      n79 = Index Array(array=w150, index=0) -> (element=w151:T11)
      n80 = Index Array(array=w147, index=0) -> (element=w148:T9)
      n81 = Or(x=w171, y=w170) -> (x .or. y?=w172:bool)
      n82 = Or(x=w159, y=w158) -> (x .or. y?=w160:bool)
      n83 = case shown="False" w172 {
        tunnel: [w213 w230] -> w177
        tunnel: w151 -> [w212 w228]
        tunnel: w175 -> [w211 w230]
        tunnel: [w210 w229] -> w166
        tunnel: w174 -> [w209 _]
        frame False {
          # "Read out each element from the data file"
          n84 = while {
            tunnel: [w224] -> w210 mode=indexing
            tunnel: w212 -> [w223]
            shift-right: [w225] -> w213
            shift-left: w211 -> [w226]
            tunnel: w209 -> [w222]
            shift-right: [w221] -> _
            shift-left: 0 -> [w220]
            stop <- w217 stop-if-true
            n85 = Read from Binary File(5:w223, 11:w226) -> (0:w215:errorcluster, 2:w224:T11, 3:w216:refnum<file>)  [unwired: 1 in, 4 out]
            n86 = Get File Position(4:w215, 7:w216) -> (2:w214:i64, 3:w225:refnum<file>)  [unwired: 1 out]
            n87 = To Long Integer(number=w214) -> (32bit integer=w221:i32)
            n88 = Greater Or Equal?(x=w221, y=w222) -> (x >= y?=w218:bool)
            n89 = Equal?(x=w221, y=w220) -> (x = y?=w219:bool)
            n90 = Or(x=w218, y=w219) -> (x .or. y?=w217:bool)
          }
        }
        frame True {
          n91 = Initialize Array(w228, 0) -> (w229:T2)
        }
      }
      n92 = case shown="False" w160 {
        tunnel: [w190 w207] -> w165
        tunnel: w148 -> [w189 w205]
        tunnel: w163 -> [w188 w207]
        tunnel: [w187 w206] -> w155
        tunnel: w162 -> [w186 _]
        frame False {
          # "Read out each element from the data file"
          n93 = while {
            tunnel: [w201] -> w187 mode=indexing
            tunnel: w189 -> [w200]
            shift-right: [w202] -> w190
            shift-left: w188 -> [w203]
            tunnel: w186 -> [w199]
            shift-right: [w198] -> _
            shift-left: 0 -> [w197]
            stop <- w194 stop-if-true
            n94 = Read from Binary File(5:w200, 11:w203) -> (0:w192:errorcluster, 2:w201:T9, 3:w193:refnum<file>)  [unwired: 1 in, 4 out]
            n95 = Get File Position(4:w192, 7:w193) -> (2:w191:i64, 3:w202:refnum<file>)  [unwired: 1 out]
            n96 = To Long Integer(number=w191) -> (32bit integer=w198:i32)
            n97 = Greater Or Equal?(x=w198, y=w199) -> (x >= y?=w195:bool)
            n98 = Equal?(x=w198, y=w197) -> (x = y?=w196:bool)
            n99 = Or(x=w195, y=w196) -> (x .or. y?=w194:bool)
          }
        }
        frame True {
          n100 = Initialize Array(w205, 0) -> (w206:T3)
        }
      }
      n101 = Close File(refnum=w177) -> ()  [unwired: 1 in, 2 out]
      n102 = Close File(refnum=w165) -> ()  [unwired: 1 in, 2 out]
    }
    frame #2 {
      n103 = local read "Procedure Name"() -> (w233:string)
      n104 = Concatenate Strings(w233, "_evp4") -> (w248:string)
      n105 = Build Path(base path=w234, name or relative path=w248) -> (appended path=w237:path)
      n106 = call <vilib>:"Open_Create_Replace File.vi"("file path"=w237) -> ("error out"=w239:errorcluster, "refnum"=w246:refnum<file>)  [unwired: 5 in, 4 out]
      n107 = Get File Size(file=w246, error in=w239) -> (refnum out=w245:refnum<file>, size (in bytes)=w243:i64, 0:w238:errorcluster)
      n108 = Unbundle By Name(w238) -> ("status"=w240:bool)
      n109 = To Long Integer(number=w243) -> (32bit integer=w244:i32)
      n110 = Equal To 0?(x=w244) -> (x = 0?=w241:bool)
      n111 = Index Array(array=w236, index=0) -> (element=w235:T12)
      n112 = Or(x=w241, y=w240) -> (x .or. y?=w242:bool)
      n113 = case shown="False" w242 {
        tunnel: [w255 w272] -> w247
        tunnel: w235 -> [w254 w269]
        tunnel: w245 -> [w253 w272]
        tunnel: [w252 w271] -> w231
        tunnel: w244 -> [w251 _]
        frame False {
          # "Read out each element from the data file"
          n114 = while {
            tunnel: [w266] -> w252 mode=indexing
            tunnel: w254 -> [w265]
            shift-right: [w267] -> w255
            shift-left: w253 -> [w268]
            tunnel: w251 -> [w264]
            shift-right: [w263] -> _
            shift-left: 0 -> [w262]
            stop <- w259 stop-if-true
            n115 = Read from Binary File(5:w265, 11:w268) -> (0:w257:errorcluster, 2:w266:T12, 3:w258:refnum<file>)  [unwired: 1 in, 4 out]
            n116 = Get File Position(4:w257, 7:w258) -> (2:w256:i64, 3:w267:refnum<file>)  [unwired: 1 out]
            n117 = To Long Integer(number=w256) -> (32bit integer=w263:i32)
            n118 = Greater Or Equal?(x=w263, y=w264) -> (x >= y?=w260:bool)
            n119 = Equal?(x=w263, y=w262) -> (x = y?=w261:bool)
            n120 = Or(x=w260, y=w261) -> (x .or. y?=w259:bool)
          }
        }
        frame True {
          n121 = Initialize Array(w269, 0) -> (w271:T5)
        }
      }
      n122 = Close File(refnum=w247) -> ()  [unwired: 1 in, 2 out]
    }
    frame #3 {
      n123 = local read "Procedure Name"() -> (w290:string)
      n124 = Concatenate Strings(w290, "_seq4") -> (w287:string)
      n125 = Build Path(base path=w276, name or relative path=w287) -> (appended path=w291:path)
      n126 = call <vilib>:"Open_Create_Replace File.vi"("file path"=w291) -> ("error out"=w278:errorcluster, "refnum"=w286:refnum<file>)  [unwired: 5 in, 4 out]
      n127 = Get File Size(file=w286, error in=w278) -> (refnum out=w285:refnum<file>, size (in bytes)=w282:i64, 0:w277:errorcluster)
      n128 = Unbundle By Name(w277) -> ("status"=w279:bool)
      n129 = To Long Integer(number=w282) -> (32bit integer=w283:i32)
      n130 = Equal To 0?(x=w283) -> (x = 0?=w280:bool)
      n131 = Index Array(array=w273, index=0) -> (element=w274:T13)
      n132 = Or(x=w280, y=w279) -> (x .or. y?=w281:bool)
      n133 = case shown="True" w281 {
        tunnel: [w297 w314] -> w289
        tunnel: w274 -> [w296 w312]
        tunnel: w285 -> [w295 w314]
        tunnel: [w294 w311] -> w284
        tunnel: w283 -> [w293 _]
        frame False {
          # "Read out each element from the data file"
          n134 = while {
            tunnel: [w308] -> w294 mode=indexing
            tunnel: w296 -> [w307]
            shift-right: [w309] -> w297
            shift-left: w295 -> [w310]
            tunnel: w293 -> [w306]
            shift-right: [w305] -> _
            shift-left: 0 -> [w304]
            stop <- w301 stop-if-true
            n135 = Read from Binary File(5:w307, 11:w310) -> (0:w299:errorcluster, 2:w308:T13, 3:w300:refnum<file>)  [unwired: 1 in, 4 out]
            n136 = Get File Position(4:w299, 7:w300) -> (2:w298:i64, 3:w309:refnum<file>)  [unwired: 1 out]
            n137 = To Long Integer(number=w298) -> (32bit integer=w305:i32)
            n138 = Greater Or Equal?(x=w305, y=w306) -> (x >= y?=w302:bool)
            n139 = Equal?(x=w305, y=w304) -> (x = y?=w303:bool)
            n140 = Or(x=w302, y=w303) -> (x .or. y?=w301:bool)
          }
        }
        frame True {
          n141 = Initialize Array(w312, 0) -> (w311:T6)
        }
      }
      n142 = Close File(refnum=w289) -> ()  [unwired: 1 in, 2 out]
    }
    frame #4 {
      n143 = local read "Procedure Name"() -> (w332:string)
      n144 = Concatenate Strings(w332, "_var4") -> (w329:string)
      n145 = Build Path(base path=w319, name or relative path=w329) -> (appended path=w333:path)
      n146 = call <vilib>:"Open_Create_Replace File.vi"("file path"=w333) -> ("error out"=w321:errorcluster, "refnum"=w328:refnum<file>)  [unwired: 5 in, 4 out]
      n147 = Get File Size(file=w328, error in=w321) -> (refnum out=w327:refnum<file>, size (in bytes)=w325:i64, 0:w320:errorcluster)
      n148 = Unbundle By Name(w320) -> ("status"=w322:bool)
      n149 = To Long Integer(number=w325) -> (32bit integer=w326:i32)
      n150 = Equal To 0?(x=w326) -> (x = 0?=w323:bool)
      n151 = Index Array(array=w316, index=0) -> (element=w317:T14)
      n152 = Or(x=w323, y=w322) -> (x .or. y?=w324:bool)
      n153 = case shown="True" w324 {
        tunnel: [w339 w356] -> w331
        tunnel: w317 -> [w338 w354]
        tunnel: w327 -> [w337 w356]
        tunnel: [w336 w353] -> w315
        tunnel: w326 -> [w335 _]
        frame False {
          # "Read out each element from the data file"
          n154 = while {
            tunnel: [w350] -> w336 mode=indexing
            tunnel: w338 -> [w349]
            shift-right: [w351] -> w339
            shift-left: w337 -> [w352]
            tunnel: w335 -> [w348]
            shift-right: [w347] -> _
            shift-left: 0 -> [w346]
            stop <- w343 stop-if-true
            n155 = Read from Binary File(5:w349, 11:w352) -> (0:w341:errorcluster, 2:w350:T14, 3:w342:refnum<file>)  [unwired: 1 in, 4 out]
            n156 = Get File Position(4:w341, 7:w342) -> (2:w340:i64, 3:w351:refnum<file>)  [unwired: 1 out]
            n157 = To Long Integer(number=w340) -> (32bit integer=w347:i32)
            n158 = Greater Or Equal?(x=w347, y=w348) -> (x >= y?=w344:bool)
            n159 = Equal?(x=w347, y=w346) -> (x = y?=w345:bool)
            n160 = Or(x=w344, y=w345) -> (x .or. y?=w343:bool)
          }
        }
        frame True {
          n161 = Initialize Array(w354, 0) -> (w353:T8)
        }
      }
      n162 = Close File(refnum=w331) -> ()  [unwired: 1 in, 2 out]
    }
    frame #5 {
      n163 = local read "Procedure Name"() -> (w374:string)
      n164 = Concatenate Strings(w374, "_srs4") -> (w372:string)
      n165 = Build Path(base path=w360, name or relative path=w372) -> (appended path=w375:path)
      n166 = call <vilib>:"Open_Create_Replace File.vi"("file path"=w375) -> ("error out"=w361:errorcluster, "refnum"=w368:refnum<file>)  [unwired: 5 in, 4 out]
      n167 = Get File Size(file=w368, error in=w361) -> (refnum out=w371:refnum<file>, size (in bytes)=w367:i64, 0:w362:errorcluster)
      n168 = Unbundle By Name(w362) -> ("status"=w363:bool)
      n169 = To Long Integer(number=w367) -> (32bit integer=w366:i32)
      n170 = Equal To 0?(x=w366) -> (x = 0?=w364:bool)
      n171 = Index Array(array=w357, index=0) -> (element=w358:T15)
      n172 = Or(x=w364, y=w363) -> (x .or. y?=w365:bool)
      n173 = case shown="False" w365 {
        tunnel: w371 -> [w380 w394]
        tunnel: [w379 w394] -> w370
        tunnel: [w378 w391] -> w369
        tunnel: w358 -> [w377 w392]
        tunnel: w366 -> [w376 _]
        frame False {
          # "Read out each element from the data file"
          n174 = while {
            tunnel: [w388] -> w378 mode=indexing
            tunnel: w377 -> [w387]
            shift-right: [w389] -> w379
            shift-left: w380 -> [w390]
            tunnel: w376 -> [w386]
            stop <- w384 stop-if-true
            n175 = Read from Binary File(5:w387, 11:w390) -> (0:w382:errorcluster, 2:w388:T15, 3:w383:refnum<file>)  [unwired: 1 in, 4 out]
            n176 = Get File Position(4:w382, 7:w383) -> (2:w381:i64, 3:w389:refnum<file>)  [unwired: 1 out]
            n177 = To Long Integer(number=w381) -> (32bit integer=w385:i32)
            n178 = Greater Or Equal?(x=w385, y=w386) -> (x >= y?=w384:bool)
          }
        }
        frame True {
          n179 = Initialize Array(w392, 0) -> (w391:T7)
        }
      }
      n180 = Close File(refnum=w370) -> ()  [unwired: 1 in, 2 out]
    }
  }
  n181 = local read "Paramaters"() -> (w22:T1)
  n182 = Bundle By Name(cluster=w22, "Master PB Staging List"=w12, "Master AO Ramp List"=w10, "Master Novatech Ramp List"=w4, "Novatech Ramps"=w7, "Sequencing Info"=w6, "SRS Ramps"=w5, "Slave PB Staging List"=w9, "Slave AO Ramp List"=w8, "Static Variables"=w1) -> (→"Paramaters":T1)
